vi "RFH-read-libreVNA.vi"(7 "file path (dialog if empty)":path, 8 "error in":errorcluster) -> (0 "error out":errorcluster, 2 "Common Format":T2)   [LabVIEW 2020, in "RFH-Reflection_File_Handler.lvlib"]
uses:
  RFH-Reflection_File_Handler.lvlib
  RFH-common_data_format.ctl
  RFH-libreVNA_data_format.ctl
panel:
  out "libreVNA data":T1
  out "string array 2":string[][](array[string])
  out "string array":string[](array[string])
  out "after substring":string
  out "text":string
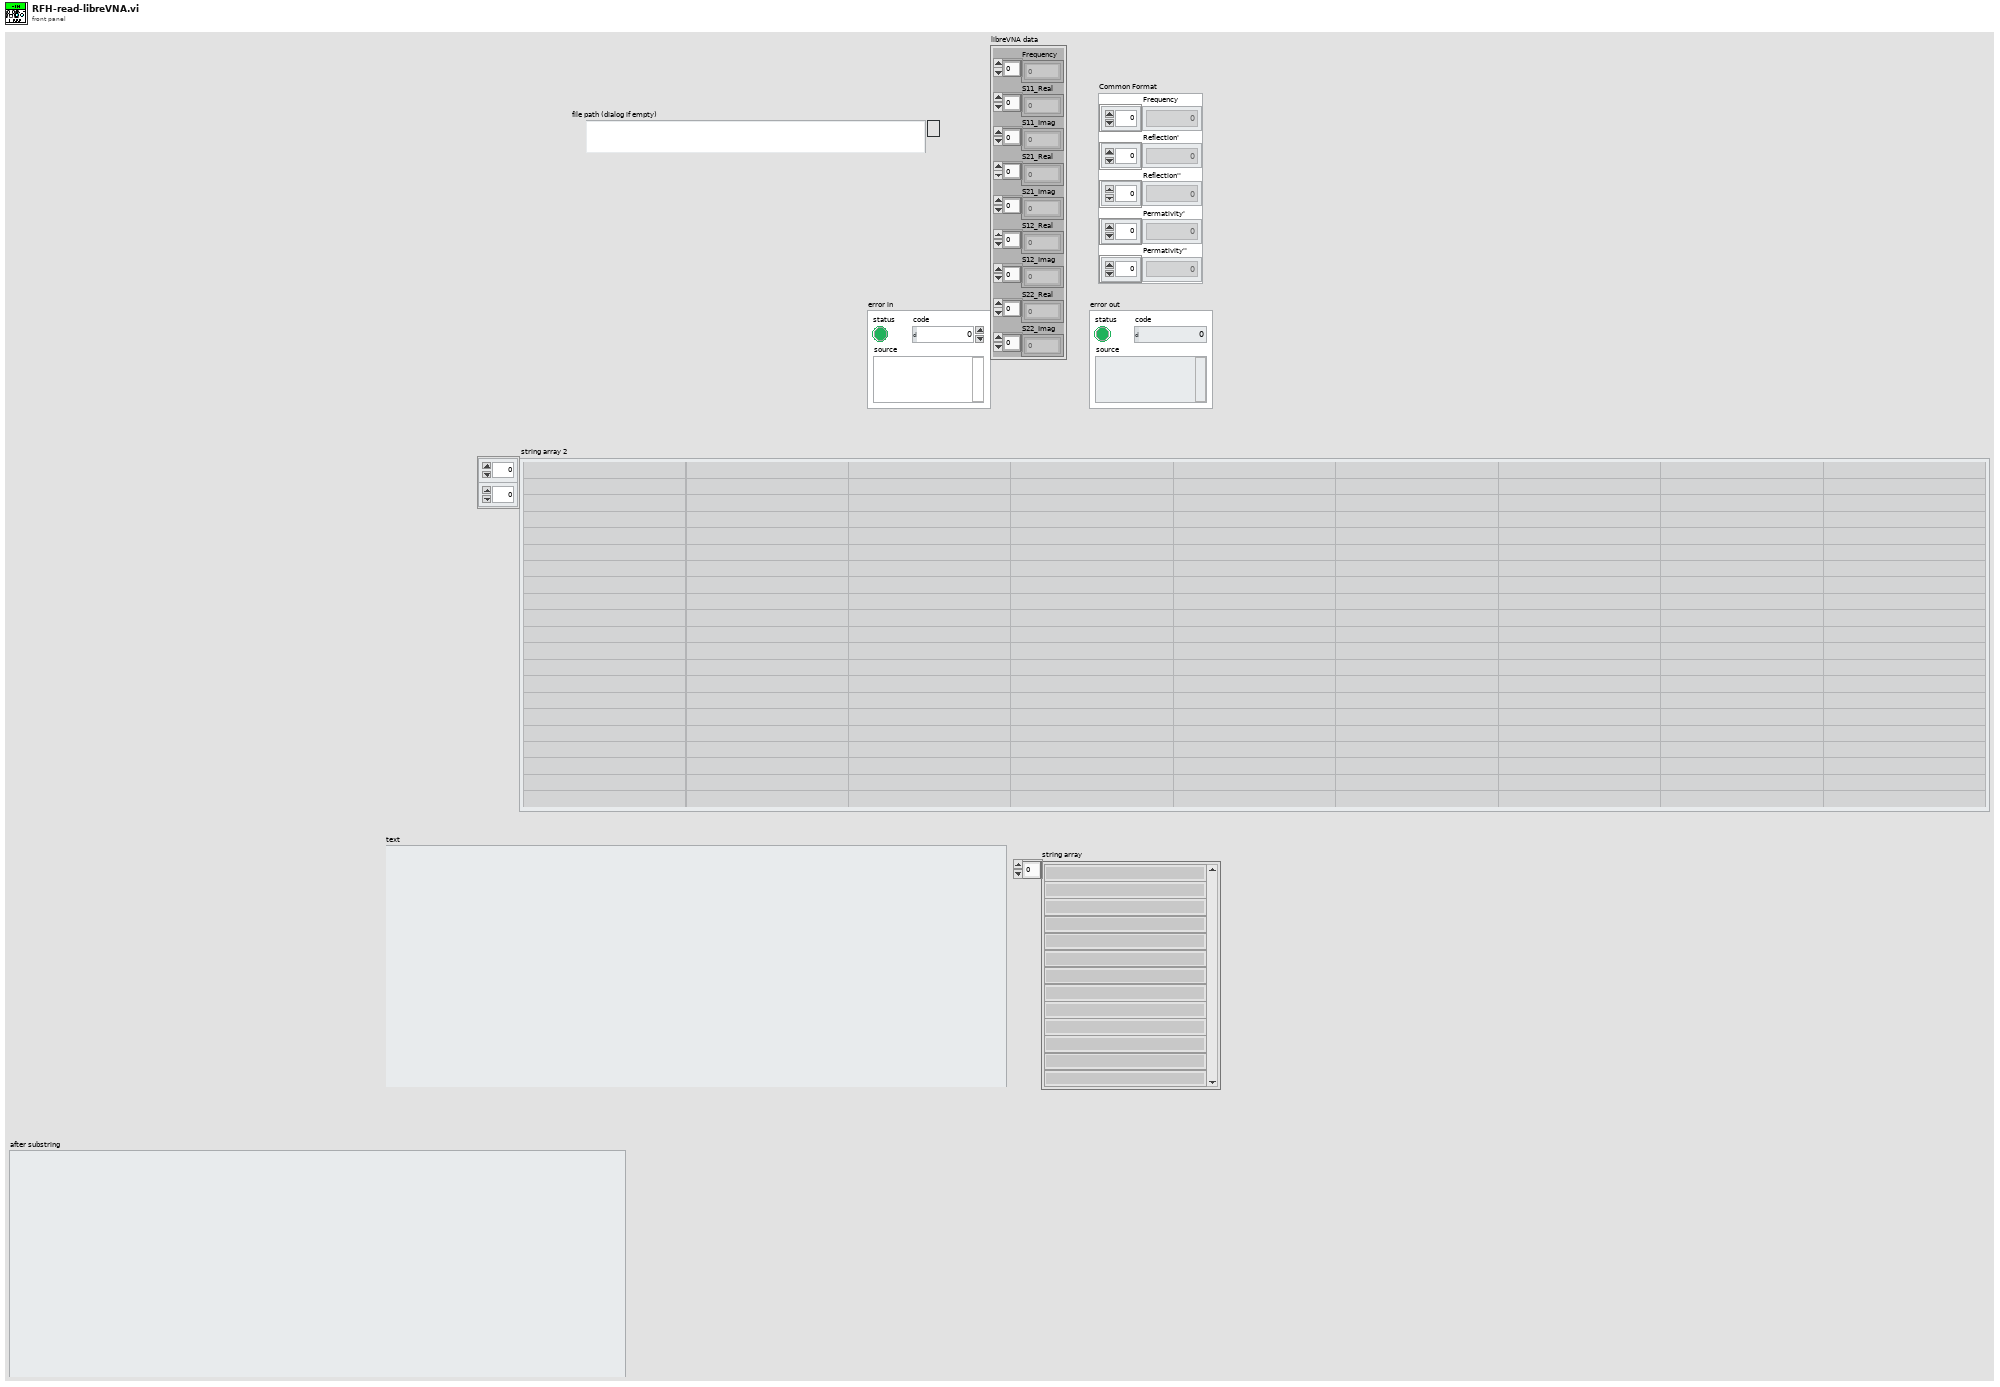
[diagram p1: front panel]
types:
  T1 = typedef "RFH-Reflection_File_Handler.lvlib/RFH-libreVNA_data_format.ctl" = cluster{"Frequency":dbl[], "S11_Real":dbl[], "S11_Imag":dbl[], "S21_Real":dbl[], "S21_Imag":dbl[], "S12_Real":dbl[], "S12_Imag":dbl[], "S22_Real":dbl[], "S22_Imag":dbl[]}
  T2 = typedef "RFH-Reflection_File_Handler.lvlib/RFH-common_data_format.ctl" = cluster{"Frequency":dbl[], "Reflection'":dbl[], "Reflection''":dbl[], "Permativity'":dbl[], "Permativity''":dbl[]}
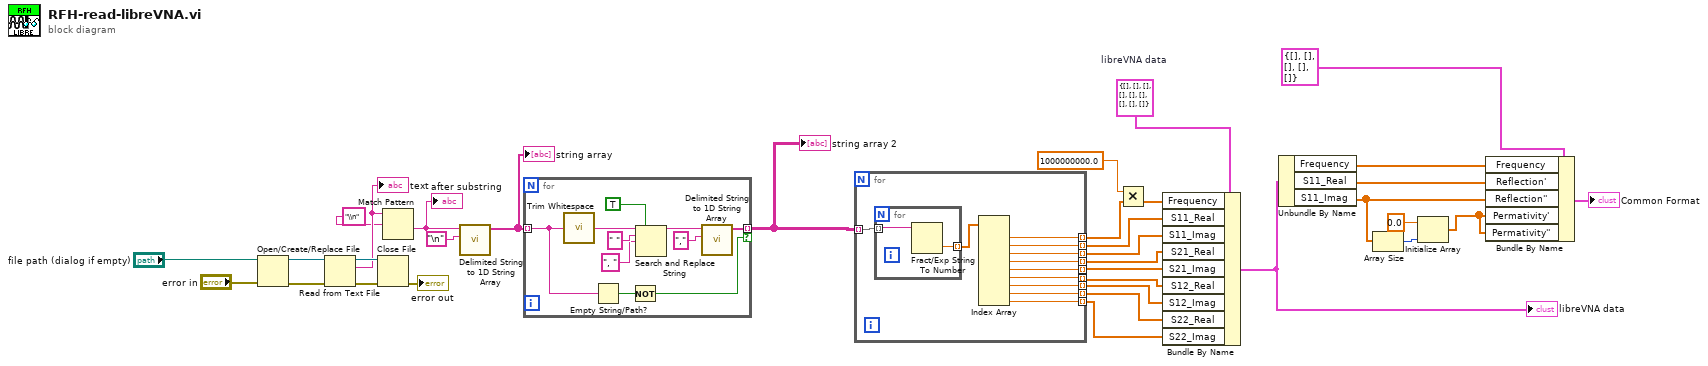
[diagram p0: block diagram]
diagram:
  w14 = T1 {"Frequency"=[], "S11_Real"=[], "S11_Imag"=[], "S21_Real"=[], "S21_Imag"=[], "S12_Real"=[], "S12_Imag"=[], "S22_Real"=[], "S22_Imag"=[]}  # libreVNA data
  n1 = Open/Create/Replace File(file path (use dialog)="file path (dialog if empty)", error in="error in") -> (refnum out=w34:refnum<file>, error out=w31:errorcluster)  [unwired: 4 in, 1 out]
  n2 = Read from Text File(file (use dialog)=w34, error in=w31) -> (refnum out=w33:refnum<file>, text=w29:string, error out=w32:errorcluster)  [unwired: 2 in, 1 out]
  "text" <- w29
  n3 = Close File(refnum=w33, error in=w32) -> (error out=→"error out":errorcluster)  [unwired: 1 out]
  n4 = Match Pattern(string=w29, regular expression="\\n" ("search string/char (-)")) -> (after substring=w25:string)  [unwired: 1 in, 3 out]
  "after substring" <- w25
  n5 = call <vilib>:"Delimited String to 1D String Array.vi"("delimiter"="\n", "delimited string"=w25) -> ("string array"=w26:string[])  [unwired: 9 in]
  "string array" <- w26
  n6 = for {
    tunnel: w26 -> [w36] mode=indexing
    tunnel: [w44] -> w24 mode=indexing if=w35
    n7 = call <vilib>:"Trim Whitespace.vi"("string"=w36) -> ("trimmed string"=w43:string)  [unwired: 1 in]
    n8 = Empty String/Path?(string/path=w36) -> (empty?=w37:bool)
    n9 = Not(x=w37) -> (.not. x?=w35:bool)
    n10 = Search and Replace String(replace all?=TRUE ("replace all? (F)"), input string=w43, search string=" ", replace string=", " ("replace string (\"\")")) -> (result string=w38:string)  [unwired: 4 in, 3 out]
    n11 = call <vilib>:"Delimited String to 1D String Array.vi"("delimiter"=",", "delimited string"=w38) -> ("string array"=w44:string[])  [unwired: 9 in]
  }
  "string array 2" <- w24
  n12 = for {
    tunnel: w24 -> [w55] mode=indexing
    tunnel: [w53] -> w23 mode=indexing
    tunnel: [w52] -> w22 mode=indexing
    tunnel: [w51] -> w21 mode=indexing
    tunnel: [w50] -> w20 mode=indexing
    tunnel: [w49] -> w19 mode=indexing
    tunnel: [w48] -> w18 mode=indexing
    tunnel: [w47] -> w17 mode=indexing
    tunnel: [w46] -> w16 mode=indexing
    tunnel: [w45] -> w15 mode=indexing
    n13 = for {
      tunnel: w55 -> [w57] mode=indexing
      tunnel: [w56] -> w54 mode=indexing
      n14 = Fract/Exp String To Number(string=w57) -> (number=w56:dbl)  [unwired: 3 in, 1 out]
    }
    n15 = Index Array(array=w54) -> (element #1=w53:dbl, element #2=w52:dbl, element #3=w51:dbl, element #4=w50:dbl, element #5=w49:dbl, element #6=w48:dbl, element #7=w47:dbl, element #8=w46:dbl, element #9=w45:dbl)  [unwired: 9 in]
  }
  n16 = Multiply(x=1000000000.0 ("element"), y=w23) -> (x*y=w11:dbl[])
  n17 = Bundle By Name(cluster=w14, "Frequency"=w11, "S11_Real"=w22, "S11_Imag"=w21, "S21_Real"=w20, "S21_Imag"=w19, "S12_Real"=w18, "S12_Imag"=w17, "S22_Real"=w16, "S22_Imag"=w15) -> (w7:T1)
  "libreVNA data" <- w7
  n18 = Unbundle By Name(w7) -> ("Frequency"=w6:dbl[], "S11_Real"=w5:dbl[], "S11_Imag"=w4:dbl[])
  n19 = Array Size(array=w4) -> (size(s)=w3:i32)
  n20 = Initialize Array(0.0 ("element"), w3) -> (w1:dbl[])
  n21 = Bundle By Name(cluster=T2 {"Frequency"=[], "Reflection'"=[], "Reflection''"=[], "Permativity'"=[], "Permativity''"=[]} ("Common Format"), "Frequency"=w6, "Reflection'"=w5, "Reflection''"=w4, "Permativity'"=w1, "Permativity''"=w1) -> (→"Common Format":T2)
